vi "BuildVIPBFile.vi"(7 "labview version":string, 8 "error in":errorcluster, 11 "path to vipb file":path) -> (0 "error out":errorcluster, 3 "build output":path)   [LabVIEW 2019]
uses:
  <vilib>/JKI/VIPM API/VIPM API_vipm_api.lvlib
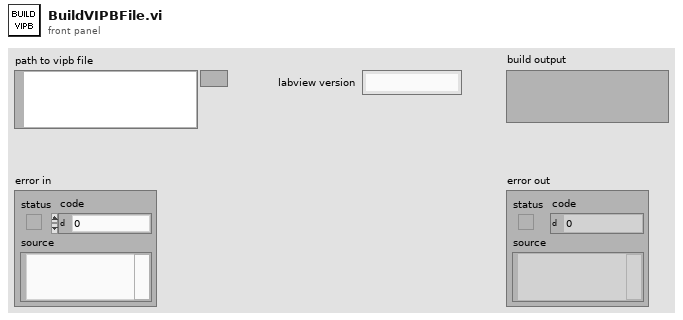
[diagram p1: front panel]
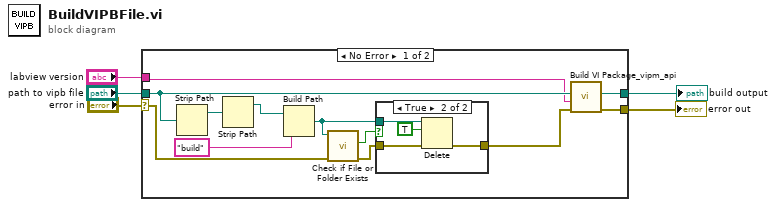
[diagram p0: block diagram]
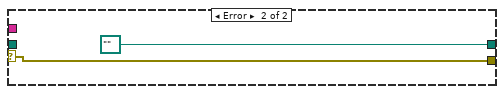
[diagram p3: hidden frame]
diagram:
  n1 = case shown="No Error" "error in" {
    selector: "error in" -> [w9 w24]
    tunnel: "path to vipb file" -> [w15 _]
    tunnel: [w17 path "" ("Build Output")] -> w4
    tunnel: [w16 w24] -> w3
    tunnel: "labview version" -> [w6 _]
    frame No Error {
      n2 = Strip Path(path=w15) -> (stripped path=w14:path)  [unwired: 1 out]
      n3 = Strip Path(path=w14) -> (stripped path=w7:path)  [unwired: 1 out]
      n4 = Build Path(base path=w7, name or relative path="build") -> (appended path=w11:path)
      n5 = call <vilib>:"Check if File or Folder Exists.vi"("error in (no error)"=w9, "path"=w11) -> ("error out"=w8:errorcluster, "file or folder exists?"=w12:bool)  [unwired: 7 in, 1 out]
      n6 = case shown="True" w12 {
        tunnel: w11 -> [_ w22]
        tunnel: w8 -> [w18 w21]
        tunnel: [w18 w20] -> w10
        frame False {
        }
        frame True {
          n7 = Delete(path (use dialog)=w22, entire hierarchy (F)=TRUE, error in=w21) -> (error out=w20:errorcluster)  [unwired: 2 in, 2 out]
        }
      }
      n8 = call <vilib>:"Build VI Package_vipm_api.vi"("error in (no error)"=w10, "LabVIEW Version"=w6, "Path to VIPB File"=w15) -> ("error out"=w16:errorcluster, "Build Output"=w17:path)  [unwired: 7 in]
    }
    frame Error {
    }
  }
  "build output" <- w4
  "error out" <- w3
